vi "PDE_Evaluate Evolut 2D Func.vi"(6 "Y":dbl[](array[numeric]), 7 "data":variant, 8 "error in (no error)":errorcluster, 9 "X":dbl[](array[numeric]), 10 "T":dbl[](array[numeric]), 11 "VIRef":refnum<vi>) -> (0 "error out":errorcluster, 3 "F(t, x, y)":dbl[][][](array[numeric]))   [LabVIEW 2017, in "NI_PDE.lvlib"]
uses:
  <vilib>/gmath/NI_PDE.lvlib
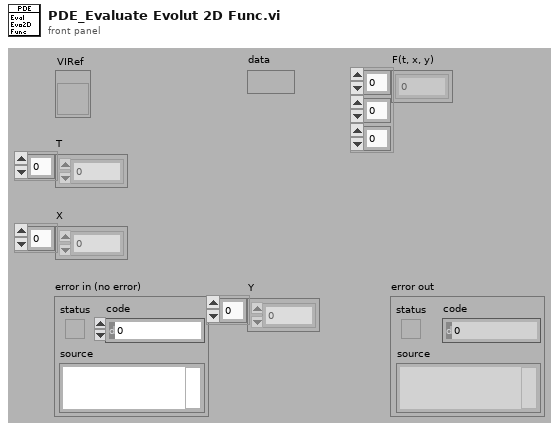
[diagram p1: front panel]
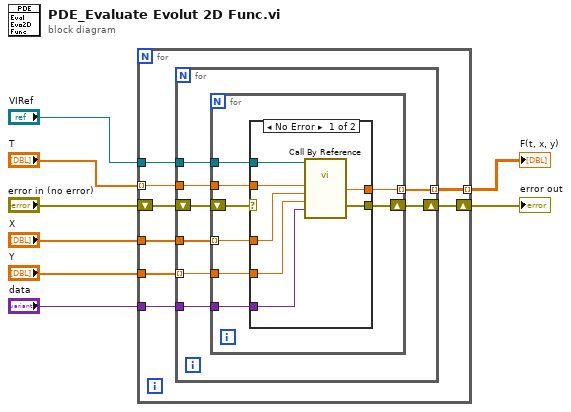
[diagram p0: block diagram]
diagram:
  n1 = for {
    tunnel: "T" -> [w14] mode=indexing
    tunnel: "X" -> [w16]
    tunnel: "VIRef" -> [w15]
    tunnel: "data" -> [w13]
    shift-right: [w12] -> w6
    shift-left: "error in (no error)" -> [w11]
    tunnel: [w10] -> w4 mode=indexing
    tunnel: "Y" -> [w9]
    n2 = for {
      tunnel: w16 -> [w24]
      tunnel: w15 -> [w23]
      tunnel: w14 -> [w22]
      tunnel: w13 -> [w21]
      tunnel: [w18] -> w10 mode=indexing
      shift-right: [w20] -> w12
      shift-left: w11 -> [w19]
      tunnel: w9 -> [w17] mode=indexing
      n3 = for {
        tunnel: w24 -> [w30] mode=indexing
        tunnel: w23 -> [w32]
        tunnel: w22 -> [w31]
        tunnel: w21 -> [w29]
        shift-right: [w28] -> w20
        shift-left: w19 -> [w27]
        tunnel: [w26] -> w18 mode=indexing
        tunnel: w17 -> [w25]
        n4 = case shown="No Error" w27 {
          selector: w27 -> [_ w40]
          tunnel: w32 -> [w39 _]
          tunnel: w31 -> [w38 _]
          tunnel: w30 -> [w37 _]
          tunnel: w29 -> [w36 _]
          tunnel: [w35 w40] -> w28
          tunnel: [w34 _] -> w26
          tunnel: w25 -> [w33 _]
          frame No Error {
            n5 = call-by-ref "?"(reference=w39, "data"=w36, "z"=w33, "y"=w37, "x"=w38) -> ("error out"=w35:errorcluster, "f(x, y, z)"=w34:dbl)  [unwired: 1 in, 2 out]
          }
          frame Error {
          }
        }
      }
    }
  }
  "F(t, x, y)" <- w4
  "error out" <- w6
